vi "Create Size by Point.vi"(8 "error in (no error)":errorcluster caption="错误输入（无错误）", 11 "Point.lvclass":refnum<class "Point.lvclass">) -> (0 "error out":errorcluster caption="错误输出", 3 "Size 输出":refnum<class "Size.lvclass"> caption="DNL_LabVIEW Object out")   [LabVIEW 2011, in "Size.lvclass"]
uses:
  Size.lvclass
  Point/Point.lvclass
panel:
  in  "Size 输入":refnum<class "Size.lvclass"> caption="DNL_LabVIEW Object in"
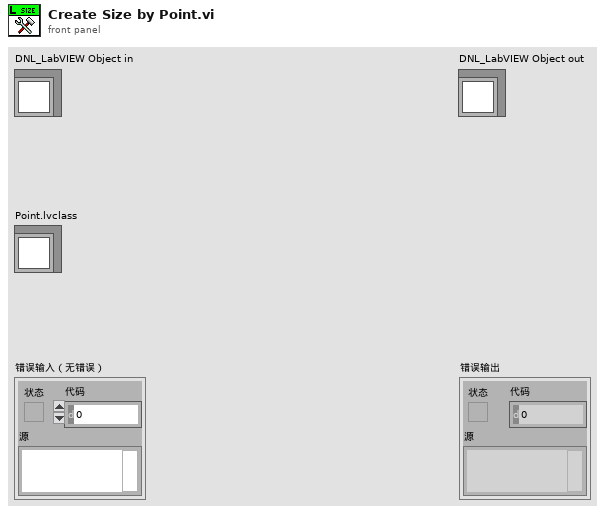
[diagram p1: front panel]
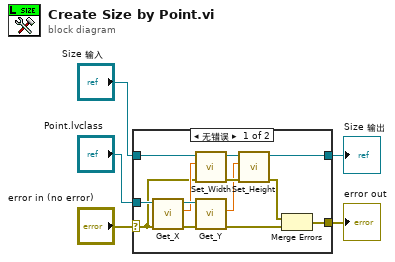
[diagram p0: block diagram]
diagram:
  n1 = case shown="无错误" "error in (no error)" {
    selector: "error in (no error)" -> [w10 w20]
    tunnel: [w6 w20] -> w4
    tunnel: [w11 w19] -> w2
    tunnel: "Size 输入" -> [w16 w19]
    tunnel: "Point.lvclass" -> [w18 _]
    frame No Error {
      n2 = call "Get_X.vi"("error in (no error)"=w10, "Point输入"=w18) -> ("error out"=w9:errorcluster, "X"=w15:dbl, "Point输出"=w17:refnum<class "Point.lvclass">)  [unwired: 7 in]
      n3 = call "Set_Width.vi"("error in (no error)"=w10, "Width"=w15, "Size输入"=w16) -> ("error out"=w13:errorcluster, "Size输出"=w14:refnum<class "Size.lvclass">)  [unwired: 7 in]
      n4 = call "Get_Y.vi"("error in (no error)"=w9, "Point输入"=w17) -> ("error out"=w7:errorcluster, "Y"=w12:dbl)  [unwired: 7 in, 1 out]
      n5 = call "Set_Height.vi"("error in (no error)"=w13, "Height"=w12, "Size输入"=w14) -> ("error out"=w8:errorcluster, "Size输出"=w11:refnum<class "Size.lvclass">)  [unwired: 7 in]
      n6 = Merge Errors(w8, w7) -> (w6:errorcluster)
    }
    frame Error {
    }
  }
  "error out" <- w4
  "Size 输出" <- w2
